vi "tm_prepare_attach_40.vi"(8 "error in (no error)":errorcluster {"code" format="%.0x"}, 9 "buffers":u64[](array[numeric]), 10 "Capture mode":i32(ring) items=["Snap", "Sequence"], 11 "Handle in":u32) -> (0 "error out":errorcluster {"code" format="%.0x"}, 3 "Handle out":u32)   [LabVIEW 2023]
uses:
  tmcamcon.dll
panel:
  out "Total Frames":i32
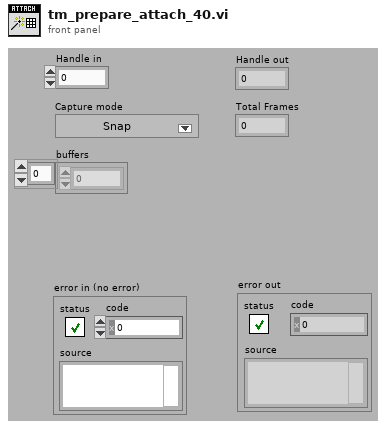
[diagram p1: front panel]
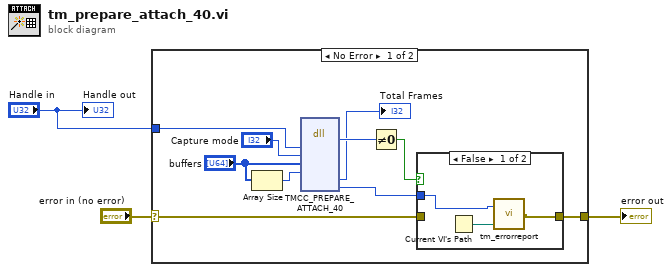
[diagram p0: block diagram]
diagram:
  n1 = case shown="No Error" "error in (no error)" {
    selector: "error in (no error)" -> [w10 w18]
    tunnel: [w7 w18] -> w1
    tunnel: "Handle in" -> [w12 _]
    frame No Error {
      n2 = Array Size(array="buffers") -> (size(s)=w5:i32)
      n3 = dll-call lib="tmcamcon.dll" fn="TMCC_PREPARE_ATTACH_40"("index"=w12, "mode"="Capture mode", "buffers"="buffers", "size"=w5) -> ("return type"=w13:u32, "totalframes"=→"Total Frames":i32, "Erval"=w9:i32)  [unwired: 9 in, 2 out]
      n4 = Not Equal To 0?(x=w13) -> (x != 0?=w8:bool)
      n5 = case shown="False" w8 {
        tunnel: w10 -> [_ w17]
        tunnel: [w14 w17] -> w7
        tunnel: w9 -> [w15 _]
        frame False {
          n6 = Current VI's Path() -> (path=w16:path)
          n7 = call "tm_errorreport.vi"("Source"=w16, "Error"=w15) -> ("error out"=w14:errorcluster)
        }
        frame True {
        }
      }
    }
    frame Error {
    }
  }
  "error out" <- w1
  "Handle out" <- "Handle in"
